vi "Configure Event Search (Serial Bus - SPI).vi"(7 "Data Width (1 Bytes)":i32=1, 8 "error in (no error)":errorcluster, 9 "Data Value (0xXX)":string="0xXX", 10 "Search Operation (0: MOSI)":i32(ring) items=["MOSI", "MISO"], 11 "VISA resource name":refnum<visa-resource-name>) -> (0 "error out":errorcluster, 3 "VISA resource name out":refnum<visa-resource-name>)   [LabVIEW 2017, in "Agilent 2000 3000 X-Series.lvlib"]
doc: "Configures the event search of SPI bus.\n\nNotes:\nThis VI is not supported by EDUX1052A/G, DSOX1202A/G, DSOX1204A/G models."
uses:
  Agilent 2000 3000 X-Series.lvlib
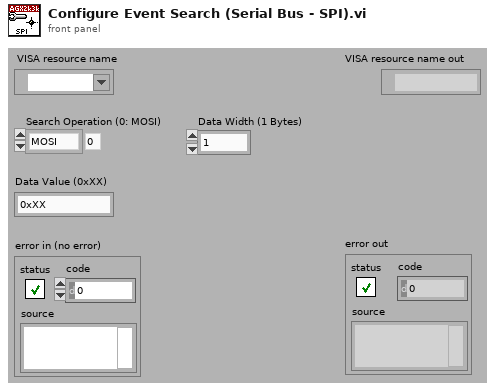
[diagram p1: front panel]
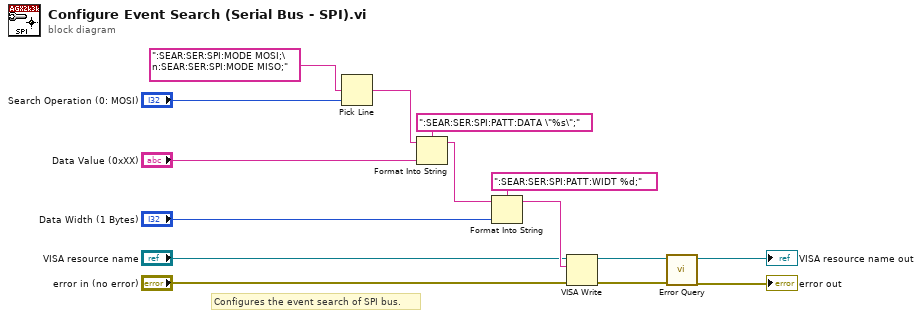
[diagram p0: block diagram]
diagram:
  # "Configures the event search of SPI bus."
  n1 = Pick Line(multi-line string=":SEAR:SER:SPI:MODE MOSI;\n:SEAR:SER:SPI:MODE MISO;", line index="Search Operation (0: MOSI)") -> (output string=w13:string)  [unwired: 1 out]
  n2 = Format Into String(format string=":SEAR:SER:SPI:PATT:DATA \"%s\";", initial string=w13, "Data Value (0xXX)") -> (resulting string=w10:string)  [unwired: 1 in, 1 out]
  n3 = Format Into String(format string=":SEAR:SER:SPI:PATT:WIDT %d;", initial string=w10, "Data Width (1 Bytes)") -> (resulting string=w7:string)  [unwired: 1 in, 1 out]
  n4 = VISA Write(VISA resource name="VISA resource name", write buffer=w7, error in (no error)="error in (no error)") -> (VISA resource name out=w4:refnum<visa-resource-name>, error out=w3:errorcluster)  [unwired: 1 out]
  n5 = call "Error Query.vi"("error in (no error)"=w3, "VISA resource name"=w4) -> ("error out"=→"error out":errorcluster, "VISA resource name out"=→"VISA resource name out":refnum<visa-resource-name>)  [unwired: 8 out]
